vi "Check If Stopped.vi"(8 "error in (no error)":errorcluster, 11 "queue in":refnum<queue>) -> (0 "error out":errorcluster, 2 "Stopped?":bool, 3 "queue out":refnum<queue>)   [LabVIEW 2010]
uses:
  RF Characterization States.ctl
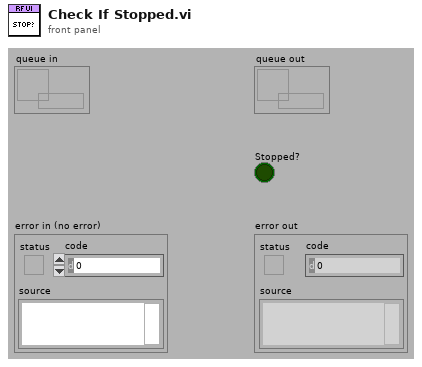
[diagram p1: front panel]
types:
  T1 = typedef "RF Characterization States.ctl" = enum16{"Initialize", "Enable/Disable Navigation", "Set Next Action", "Set Prev Action", "Set Stop Action", "Prev Action Triggered", "Next Action Triggered", "Stop Action Triggered", "Move Gantry to Position", "Display Configuration Tab", "Check Configuration", "Display Attenuation Tab", "Check Attenuation Config", "Start Attenuation Test", "Check Attenuation Results", "Display Power Tab", "Check Power Config", "Start Power Test", "Check Power Results", "Display Mapping Tab", "Check Mapping Config", "Start Mapping Test", "Take Mapping Sample", "Finish Mapping Test", "Check Mapping Results", "Display Report Tab", "Generate Report", "Save Report", "Error", "Shutdown"}
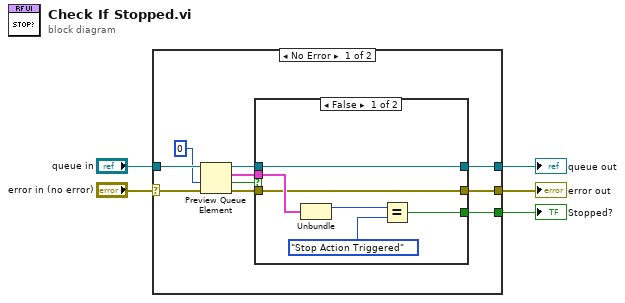
[diagram p0: block diagram]
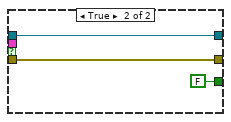
[diagram p2: hidden frame]
diagram:
  n1 = case shown="No Error" "error in (no error)" {
    selector: "error in (no error)" -> [w15 w26]
    tunnel: "queue in" -> [w14 w25]
    tunnel: [w10 w25] -> w1
    tunnel: [w7 _] -> w3
    tunnel: [w6 w26] -> w2
    frame No Error {
      n2 = Preview Queue Element(queue=w14, timeout in ms (-1)=0, error in (no error)=w15) -> (queue out=w9:refnum<queue>, element=w8:cluster{"State":T1, "Data":variant}, timed out?=w12:bool, error out=w11:errorcluster)
      n3 = case shown="False" w12 {
        tunnel: w11 -> [w16 w22]
        tunnel: [w21 w23] -> w10
        tunnel: w9 -> [w21 w23]
        tunnel: w8 -> [w20 _]
        tunnel: [w17 FALSE] -> w7
        tunnel: [w16 w22] -> w6
        frame False {
          n4 = Unbundle(w20) -> ("State"=w19:T1)  [unwired: 1 out]
          n5 = Equal?(x=w19, y=RF_Characterization_States."Stop Action Triggered" ("x")) -> (x = y?=w17:bool)
        }
        frame True {
        }
      }
    }
    frame Error {
    }
  }
  "error out" <- w2
  "Stopped?" <- w3
  "queue out" <- w1
